vi "Day 11.vi"() -> ()   [LabVIEW 2023]
uses:
  <vilib>/Utility/error.llb/Trim Whitespace One-Sided.vi
panel:
  out "Monkeys":T1(array[cluster])
  out "Answer 1":i32
  in  "test":bool
  in  "test input":string="Monkey 0:\n  Starting items: 79, 98\n  Operation: new = old * 19\n  Test: divisible by 23\n    If true: throw to monkey 2\n    If false: throw to monkey 3\n\nMonkey 1:\n  Starting items: 54, 65, 75, 74\n  Operation: new = old + 6\n  Test: divisible by 19\n    If true: throw to monkey 2\n    If false: throw to monkey 0\n\nMonkey 2:\n  Starting items: 79, 60, 97\n  Operation: new = old * old\n  Test: divisible by 13\n    If true: throw to monkey 1\n    If false: throw to monkey 3\n\nMonkey 3:\n  Starting items: 74\n  Operation: new = old + 3\n  Test: divisible by 17\n    If true: throw to monkey 0\n    If false: throw to monkey 1"
  in  "input":string="Monkey 0:\n  Starting items: 57, 58\n  Operation: new = old * 19\n  Test: divisible by 7\n    If true: throw to monkey 2\n    If false: throw to monkey 3\n\nMonkey 1:\n  Starting items: 66, 52, 59, 79, 94, 73\n  Operation: new = old + 1\n  Test: divisible by 19\n    If true: throw to monkey 4\n    If false: throw to monkey 6\n\nMonkey 2:\n  Starting items: 80\n  Operation: new = old + 6\n  Test: divisible by 5\n    If true: throw to monkey 7\n    If false: throw to monkey 5\n\nMonkey 3:\n  Starting items: 82, 81, 68, 66, 71, 83, 75, 97\n  Operation: new = old + 5\n  Test: divisible by 11\n    If true: throw to monkey 5\n    If false: throw to monkey 2\n\nMonkey 4:\n  Starting items: 55, 52, 67, 70, 69, 94, 90\n  Operation: new = old * old\n  Test: divisible by 17\n    If true: throw to monkey 0\n    If false: throw to monkey 3\n\nMonkey 5:\n  Starting items: 69, 85, 89, 91\n  Operation: new = old + 7\n  Test: divisible by 13\n    If true: throw to monkey 1\n    If false: throw to monkey 7\n\nMonkey 6:\n  Starting items: 75, 53, 73, 52, 75\n  Operation: new = old * 7\n  Test: divisible by 2\n    If true: throw to monkey 0\n    If false: throw to monkey 4\n\nMonkey 7:\n  Starting items: 94, 60, 79\n  Operation: new = old + 2\n  Test: divisible by 3\n    If true: throw to monkey 1\n    If false: throw to monkey 6\n"
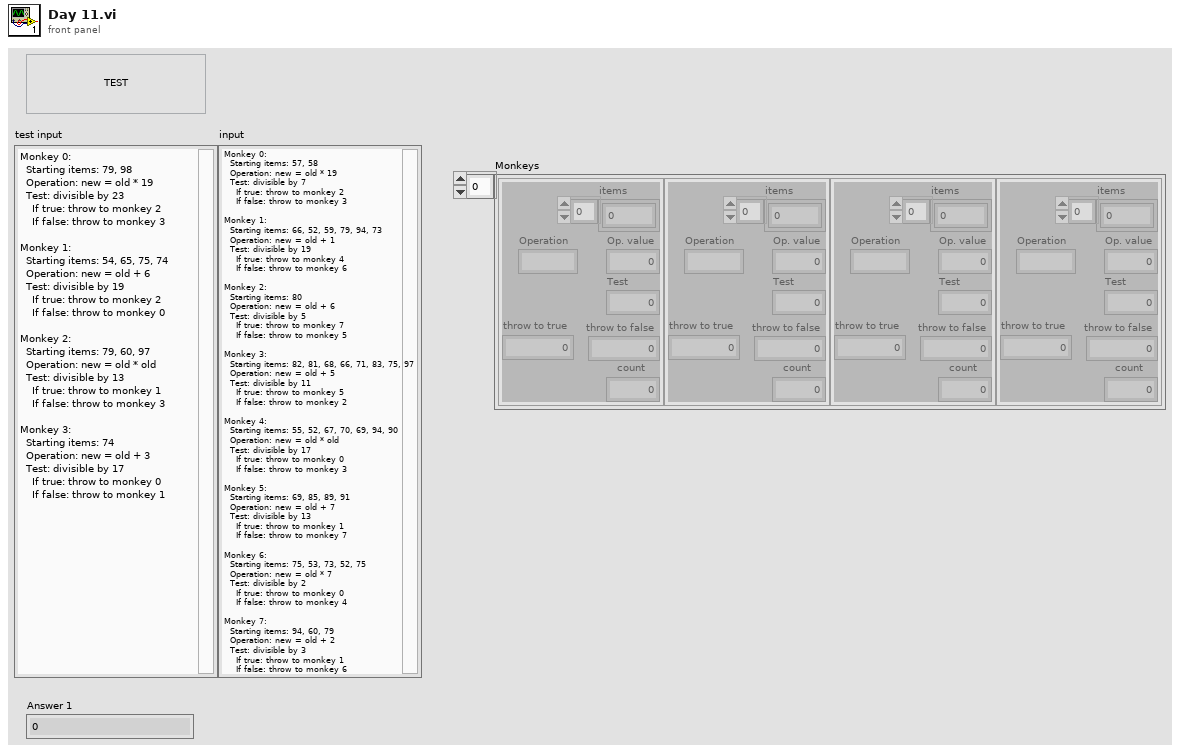
[diagram p1: front panel]
types:
  T1 = cluster{"items":i32[], "Operation":string, "Op. value":i32, "throw to true":i32, "throw to false":i32, "Test":i32, "count":i32}[]
  T2 = cluster{"items":i32[], "Operation":string, "Op. value":i32, "throw to true":i32, "throw to false":i32, "Test":i32, "count":i32}
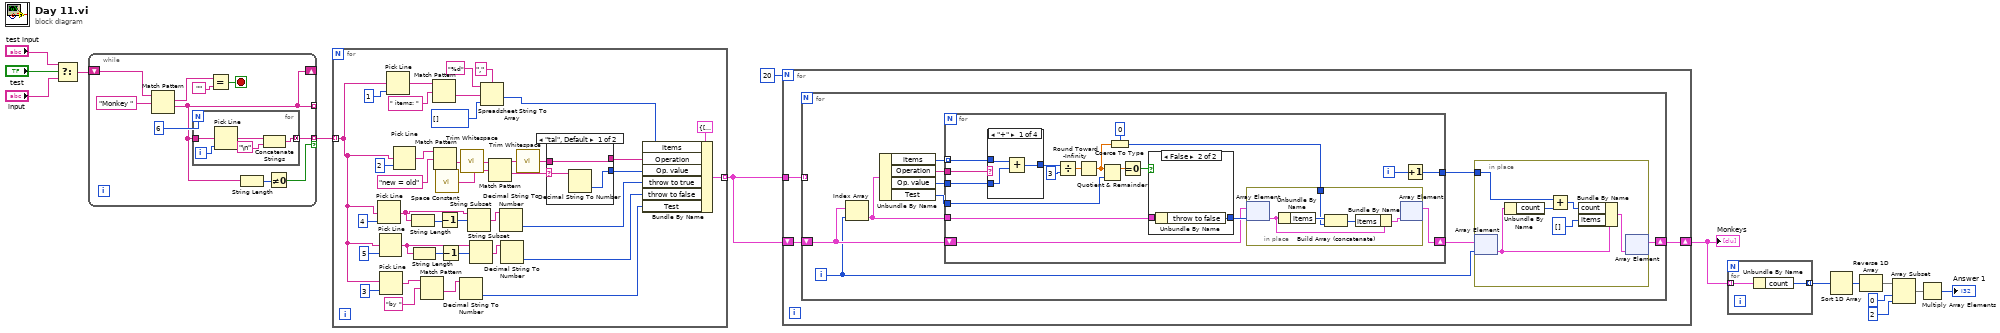
[diagram p0: block diagram]
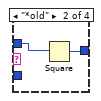
[diagram p2: hidden frame]
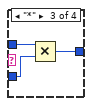
[diagram p3: hidden frame]
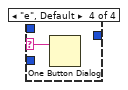
[diagram p4: hidden frame]
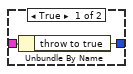
[diagram p5: hidden frame]
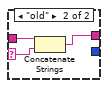
[diagram p6: hidden frame]
diagram:
  n1 = Select(t="test input", s="test", f="input") -> (s? t:f=w11:string)
  n2 = while {
    shift-right: [w16] -> _
    shift-left: w11 -> [w25]
    tunnel: [w18] -> w12 mode=indexing if=w17
    tunnel: [w16] -> _ mode=indexing
    stop <- w20 stop-if-true
    n3 = Match Pattern(string=w25, regular expression="Monkey ") -> (match substring=w21:string, after substring=w16:string)  [unwired: 1 in, 2 out]
    n4 = for {
      N: 6 -> [_]
      tunnel: w16 -> [w30]
      tunnel: [w27] -> w18 mode=concatenating
      i -> [w28]
      n5 = Pick Line(multi-line string=w30, line index=w28) -> (output string=w29:string)  [unwired: 1 in]
      n6 = Concatenate Strings(w29, "\n") -> (w27:string)
    }
    n7 = Equal?(x=w21, y="") -> (x = y?=w20:bool)
    n8 = String Length(string=w16) -> (length=w19:i32)
    n9 = Not Equal To 0?(x=w19) -> (x != 0?=w17:bool)
  }
  n10 = for {
    tunnel: w12 -> [w35] mode=indexing
    tunnel: [w61] -> w9 mode=indexing
    n11 = Pick Line(multi-line string=w35, line index=4) -> (output string=w44:string)  [unwired: 1 in]
    n12 = Pick Line(multi-line string=w35, line index=5) -> (output string=w46:string)  [unwired: 1 in]
    n13 = Pick Line(multi-line string=w35, line index=3) -> (output string=w39:string)  [unwired: 1 in]
    n14 = Pick Line(multi-line string=w35, line index=1) -> (output string=w67:string)  [unwired: 1 in]
    n15 = Pick Line(multi-line string=w35, line index=2) -> (output string=w59:string)  [unwired: 1 in]
    n16 = String Length(string=w44) -> (length=w51:i32)
    n17 = String Length(string=w46) -> (length=w47:i32)
    n18 = Match Pattern(string=w39, regular expression="by ") -> (after substring=w38:string)  [unwired: 1 in, 3 out]
    n19 = Match Pattern(string=w67, regular expression=" items: ") -> (after substring=w65:string)  [unwired: 1 in, 3 out]
    n20 = Match Pattern(string=w59, regular expression="new = old") -> (after substring=w57:string)  [unwired: 1 in, 3 out]
    n21 = call <vilib>:"Space Constant.vi"() -> ("String"=w56:string)
    n22 = Decrement(x=w51) -> (x-1=w42:i32)
    n23 = Decrement(x=w47) -> (x-1=w41:i32)
    n24 = Decimal String To Number(string=w38) -> (number=w37:i32)  [unwired: 2 in, 1 out]
    n25 = call <vilib>:"Trim Whitespace.vi"("string"=w57) -> ("trimmed string"=w55:string)  [unwired: 1 in]
    n26 = String Subset(string=w44, offset (0)=w42) -> (substring=w50:string)  [unwired: 1 in]
    n27 = String Subset(string=w46, offset (0)=w41) -> (substring=w48:string)  [unwired: 1 in]
    n28 = Spreadsheet String To Array(delimiter (Tab)="," ("format string"), format string="%d", spreadsheet string=w65, array type (2D Dbl)=i32[] [] ("output array")) -> (array=w62:i32[])
    n29 = Match Pattern(string=w55, regular expression=w56) -> (before substring=w54:string, after substring=w34:string)  [unwired: 1 in, 2 out]
    n30 = Decimal String To Number(string=w50) -> (number=w49:i32)  [unwired: 2 in, 1 out]
    n31 = Decimal String To Number(string=w48) -> (number=w43:i32)  [unwired: 2 in, 1 out]
    n32 = call <vilib>:"Trim Whitespace.vi"("string"=w54) -> ("trimmed string"=w33:string)  [unwired: 1 in]
    n33 = case shown="\"tal\", Default" w34 {
      selector: w34 -> [w71 w74]
      tunnel: [w72 _] -> w53
      tunnel: w33 -> [w70 w75]
      tunnel: [w70 w73] -> w32
      frame "tal", Default {
        n34 = Decimal String To Number(string=w71) -> (number=w72:i32)  [unwired: 2 in, 1 out]
      }
      frame "old" {
        n35 = Concatenate Strings(w75, w74) -> (w73:string)
      }
    }
    n36 = Bundle By Name(cluster=T2 {"items"=[79, 98], "Operation"="*", "Op. value"=19, "throw to true"=2, "throw to false"=3, "Test"=23, "count"=0} ("input cluster"), "items"=w62, "Operation"=w32, "Op. value"=w53, "throw to true"=w49, "throw to false"=w43, "Test"=w37) -> (w61:T2)
  }
  n37 = for {
    N: 20 -> [_]
    tunnel: w9 -> [w78]
    shift-right: [w77] -> w8
    shift-left: w9 -> [w76]
    n38 = for {
      tunnel: w78 -> [_] mode=indexing
      shift-right: [w81] -> w77
      shift-left: w76 -> [w83]
      i -> [w79]
      n39 = Index Array(array=w83, index=w79) -> (element=w84:T2)
      n40 = Unbundle By Name(w84) -> ("items"=w88:i32[], "Operation"=w87:string, "Op. value"=w86:i32, "Test"=w85:i32)
      n41 = for {
        tunnel: w88 -> [w105] mode=indexing
        tunnel: w87 -> [w106]
        tunnel: w86 -> [w104]
        tunnel: w85 -> [w100]
        tunnel: w84 -> [w97]
        shift-right: [w92] -> w82
        shift-left: w83 -> [w91]
        tunnel: [w89] -> w80
        i -> [w90]
        n42 = case shown="\"+\"" w106 {
          selector: w106 -> [_ _ _ w115]
          tunnel: w105 -> [w108 w110 w114 _]
          tunnel: w104 -> [w107 _ w113 _]
          tunnel: [w109 w111 w112 _] -> w103
          frame "+" {
            n43 = Add(x=w108, y=w107) -> (x+y=w109:i32)
          }
          frame "*old" {
            n44 = Square(x=w110) -> (x^2=w111:i32)
          }
          frame "*" {
            n45 = Multiply(x=w114, y=w113) -> (x*y=w112:i32)
          }
          frame "e", Default {
            n46 = One Button Dialog(message=w115) -> ()  [unwired: 1 in, 1 out]
          }
        }
        n47 = Divide(x=w103, y=3) -> (x/y=w101:dbl)
        n48 = Round Toward -Infinity(1:w101) -> (0:w96:dbl)
        n49 = Quotient & Remainder(x=w96, y=w100) -> (x-y*floor(x/y)=w99:dbl)  [unwired: 1 out]
        n50 = Coerce To Type(0:w96, 1:0 ("y")) -> (2:w94:i32)
        n51 = Equal To 0?(x=w99) -> (x = 0?=w98:bool)
        n52 = case shown="False" w98 {
          tunnel: w97 -> [w122 w124]
          tunnel: [w121 w123] -> w93
          frame True {
            n53 = Unbundle By Name(w122) -> ("throw to true"=w121:i32)
          }
          frame False {
            n54 = Unbundle By Name(w124) -> ("throw to false"=w123:i32)
          }
        }
        n55 = in-place {
          in-place-border: w94 -> [w118]
          n56 = in-place-array #1(w91, w93) -> (w116:T2)
          n57 = Unbundle By Name(w116) -> ("items"=w119:i32[])
          n58 = Build Array (concatenate)(w119, w118) -> (w120:i32[])
          n59 = Bundle By Name(cluster=w116, "items"=w120) -> (w117:T2)
          n60 = in-place-array #1(w117) -> (w92:T1)  [unwired: 1 out]
        }
        n61 = Increment(x=w90) -> (x+1=w89:i32)
      }
      n62 = in-place {
        in-place-border: w80 -> [w125]
        n63 = in-place-array #2(w82, w79) -> (w128:T2)
        n64 = Unbundle By Name(w128) -> ("count"=w127:i32)
        n65 = Add(x=w125, y=w127) -> (x+y=w126:i32)
        n66 = Bundle By Name(cluster=w128, "count"=w126, "items"=i32[] []) -> (w130:T2)
        n67 = in-place-array #2(w130) -> (w81:T1)  [unwired: 1 out]
      }
    }
  }
  "Monkeys" <- w8
  n68 = for {
    tunnel: w8 -> [w132] mode=indexing
    tunnel: [w131] -> w7 mode=indexing
    n69 = Unbundle By Name(w132) -> ("count"=w131:i32)
  }
  n70 = Sort 1D Array(array=w7) -> (sorted array=w6:i32[])
  n71 = Reverse 1D Array(array=w6) -> (reversed array=w5:i32[])
  n72 = Array Subset(array=w5, index=0, length=2) -> (w2:i32[])
  n73 = Multiply Array Elements(1:w2) -> (0:→"Answer 1":i32)
